vi "Neko_diagonal.vi"() -> ()   [LabVIEW 2023]
panel:
  out "Ring":u16(ring)
  in  "stop":bool
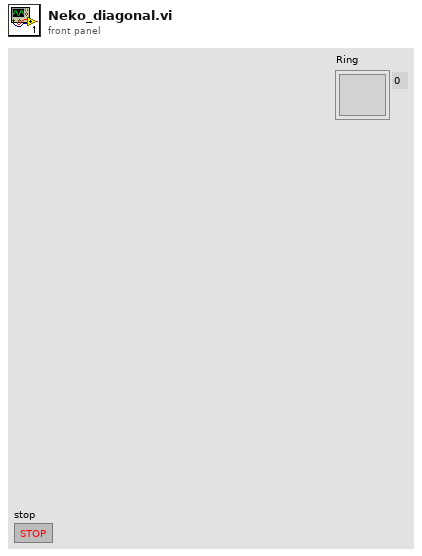
[diagram p1: front panel]
types:
  T1 = typedef "LVPoint32TypeDef.ctl" = cluster{"Horizontal":i32, "Vertical":i32}
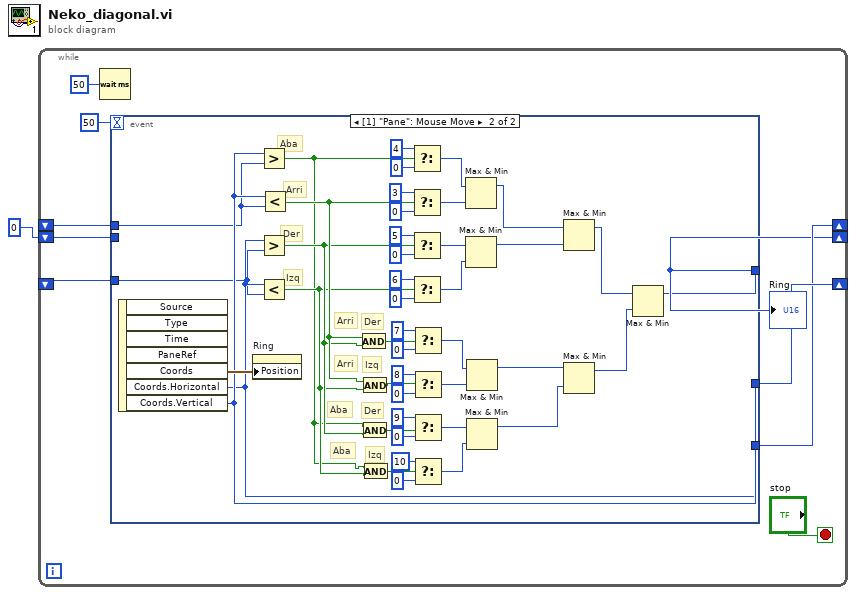
[diagram p0: block diagram]
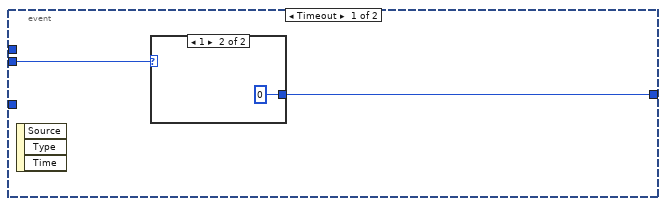
[diagram p2: hidden frame]
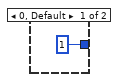
[diagram p3: hidden frame]
diagram:
  n1 = while {
    shift-right: [w2] -> _
    shift-left: 0 -> [w8]
    shift-right: [w6] -> _
    shift-left: _ -> [w5]
    shift-right: [w4] -> _
    shift-left: _ -> [w3]
    stop <- "stop" stop-if-true
    n2 = Wait (ms)(milliseconds to wait=50) -> ()  [unwired: 1 out]
    n3 = event shown="[1] \"Pane\": Mouse Move" {
      selector: _ -> [_ _]
      dyn-events: _ -> [_ _]
      timeout: 50 -> [_ _]
      tunnel: w8 -> [w12 _]
      tunnel: [_ w43] -> w6
      tunnel: w5 -> [_ w42]
      tunnel: [_ w49] -> w4
      tunnel: w3 -> [_ w48]
      tunnel: [w11 w23] -> w2
      event Timeout {
        n4 = event-data() -> ()  [unwired: 1 in, 3 out]
        n5 = case shown="1" w12 {
          tunnel: [1 0] -> w11
          frame 0, Default {
          }
          frame 1 {
          }
        }
      }
      event Mouse Move {
        # "Aba"
        # "Aba"
        # "Izq"
        # "Der"
        # "Izq"
        # "Der"
        # "Arri"
        # "Arri"
        # "Izq"
        # "Aba"
        # "Der"
        # "Arri"
        n6 = event-data() -> ("Coords"=w58:T1, "Coords.Horizontal"=w43:i32, "Coords.Vertical"=w49:i32)  [unwired: 1 in, 4 out]
        n7 = property on="Ring" class="Ring (strict)"("Position"=w58) -> ()  [unwired: 2 in, 2 out]
        n8 = Greater?(x=w49, y=w48) -> (0:w16:bool)
        n9 = Greater?(x=w43, y=w42) -> (0:w19:bool)
        n10 = Less?(x=w43, y=w42) -> (x < y?=w17:bool)
        n11 = Less?(x=w49, y=w48) -> (x < y?=w21:bool)
        n12 = And(x=w21, y=w19) -> (x .and. y?=w22:bool)
        n13 = And(x=w21, y=w17) -> (x .and. y?=w20:bool)
        n14 = And(x=w16, y=w19) -> (x .and. y?=w18:bool)
        n15 = And(x=w16, y=w17) -> (x .and. y?=w15:bool)
        n16 = Select(t=4, s=w16, f=0) -> (s? t:f=w45:i32)
        n17 = Select(t=3, s=w21, f=0) -> (s? t:f=w44:i32)
        n18 = Select(t=5, s=w19, f=0) -> (s? t:f=w47:i32)
        n19 = Select(t=6, s=w17, f=0) -> (s? t:f=w46:i32)
        n20 = Select(t=7, s=w22, f=0) -> (s? t:f=w32:i32)
        n21 = Select(t=8, s=w20, f=0) -> (s? t:f=w31:i32)
        n22 = Select(t=9, s=w18, f=0) -> (s? t:f=w34:i32)
        n23 = Select(t=10, s=w15, f=0) -> (s? t:f=w33:i32)
        n24 = Max & Min(x=w45, y=w44) -> (max(x,y)=w29:i32)  [unwired: 1 out]
        n25 = Max & Min(x=w47, y=w46) -> (max(x,y)=w28:i32)  [unwired: 1 out]
        n26 = Max & Min(x=w32, y=w31) -> (max(x,y)=w27:i32)  [unwired: 1 out]
        n27 = Max & Min(x=w34, y=w33) -> (max(x,y)=w26:i32)  [unwired: 1 out]
        n28 = Max & Min(x=w29, y=w28) -> (max(x,y)=w25:i32)  [unwired: 1 out]
        n29 = Max & Min(x=w27, y=w26) -> (max(x,y)=w24:i32)  [unwired: 1 out]
        n30 = Max & Min(x=w25, y=w24) -> (max(x,y)=w23:i32)  [unwired: 1 out]
      }
    }
    "Ring" <- w2
  }
